vi "XiXi-1(Multify And Boolean).vi"(10 "X[-1]":bool, 11 "Xi":bool[](array[boolean])) -> (3 "Yi":bool[](array[boolean]))   [LabVIEW 2012]
doc: "Calculate sums of consecutive array elements. 0th element of output is equal to x(0)+ x(-1), where x(-1) is an optional scalar input that defaults to zero."
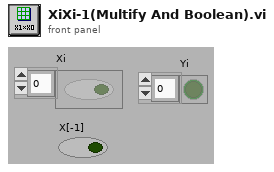
[diagram p1: front panel]
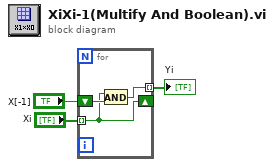
[diagram p0: block diagram]
diagram:
  n1 = for {
    shift-right: [w5] -> _
    shift-left: "X[-1]" -> [w6]
    tunnel: "Xi" -> [w5] mode=indexing
    tunnel: [w4] -> w1 mode=indexing
    n2 = And(x=w5, y=w6) -> (x .and. y?=w4:bool)
  }
  "Yi" <- w1
